vi "CFG File Editor.vi"(0 "Parameters In":T1[](array[typedef]), 11 "error in (no error)":errorcluster) -> (4 "Parameters Out":T1[](array[typedef]), 8 "Cancelled":bool, 15 "error out":errorcluster)   [LabVIEW 2012]
uses:
  Type Defs/CFG Key Cluster.ctl
  Type Defs/CFG Tag Type Enum.ctl
panel:
  in  "DAQmx Terminal":tag
  in  "DAQmx Channel":tag
  in  "Exit":bool
  in  "I32":i32
  in  "VISA resource name":refnum<visa-resource-name>
  in  "VISA Rsrc":refnum<visa-resource-name>
  in  "String":string
  in  "Ring":u16(ring) items=["Yaw/Brake ATP", "Yaw/Brake Integration/Endurance", "Pitch/Roll ATP", "Pitch/Roll Integration/Endurance", "Control Stand"]
  in  "Path":path
  in  "BOOL":bool
  in  "DBL":dbl min=1.0 max=160.0 step=1.0
  in  "Cancel":bool
  out "Status":string="Initialize"
  in  "Tree":string(tree)
  # "Configuration"
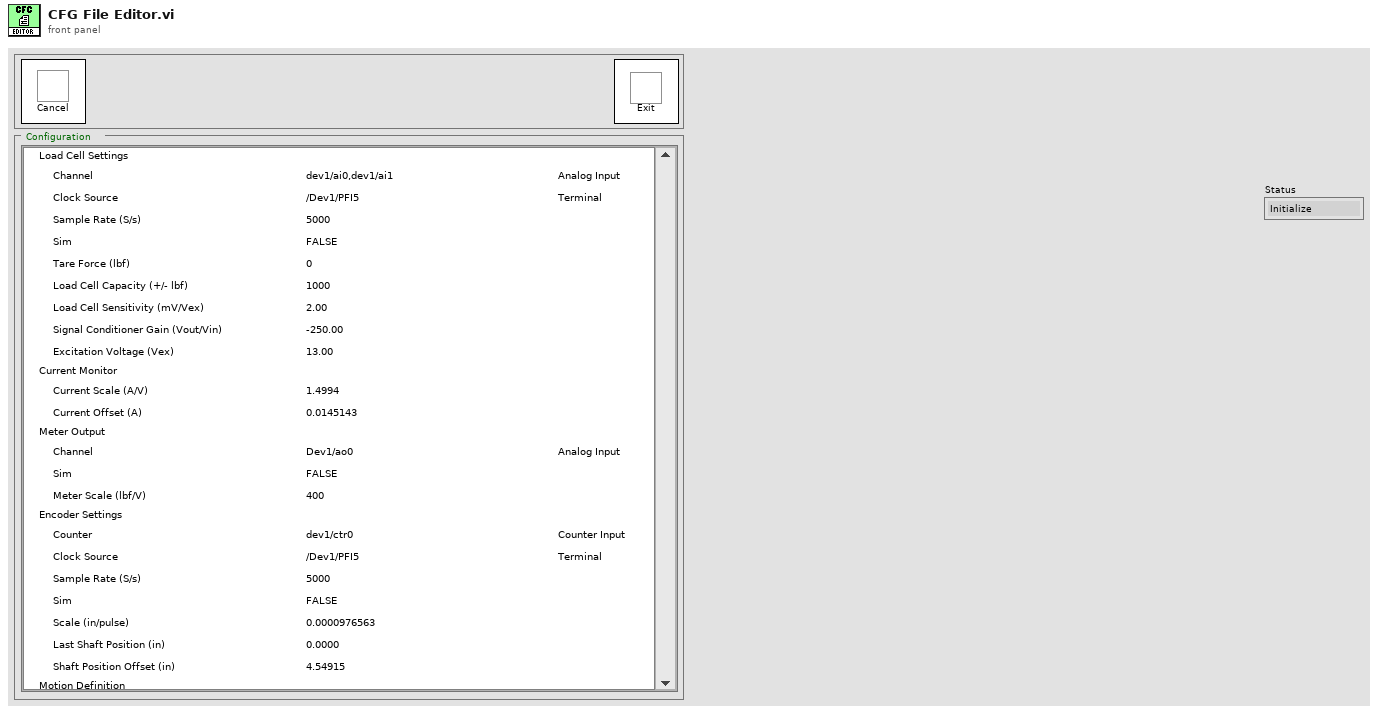
[diagram p1: front panel]
types:
  T1 = typedef "CFG Key Cluster.ctl" = cluster{"Strings []":string[], "Disabled Items []":i32[], "Value":variant, "Format String":string, "Tag":string, "Type":T2, "Section":string, " Ctl Ref":refnum<vi>, "Data Range":cluster{"Minimum":dbl, "Maximum":dbl, "Increment":dbl}, "Unit":string, "Special Instructions":string, "Delimiter(s)":string, "Dimensions":i32, "Element Type":T2, "Array Value String":string}
  T2 = typedef "CFG Tag Type Enum.ctl" = enum16{"Digital", "Slide", "Enum", "Boolean", "String", "Path", "Array", "VISAResourceName", "DAQmxName", "Cluster"}
  T3 = enum32{"existing file", "new file", "new or existing file", "existing dir", "new dir", "new or existing dir", "existing file (use LLBs)", "new file (use LLBs)", "new or existing file (use LLBs)", "new or existing file or directory (use LLBs)", "existing dir (use LLBs)", "new dir (use LLBs)", "new or existing dir (use LLBs)", "existing file or dir", "new file or dir", "new or existing file or dir", "existing file or dir (use LLBs)", "new file or dir (use LLBs)"}
  T4 = cluster{"Minimum":dbl, "Maximum":dbl, "Increment":dbl}
  T5 = typedef "LVPositionTypeDef.ctl" = cluster{"Left":i32, "Top":i32}
  T6 = typedef "CFG DAQmx Type Enum.ctl" = enum16{"Analog Input", "Analog Output", "Digital Input", "Digital Output", "Counter Input", "Counter Output", "Terminal", ""}
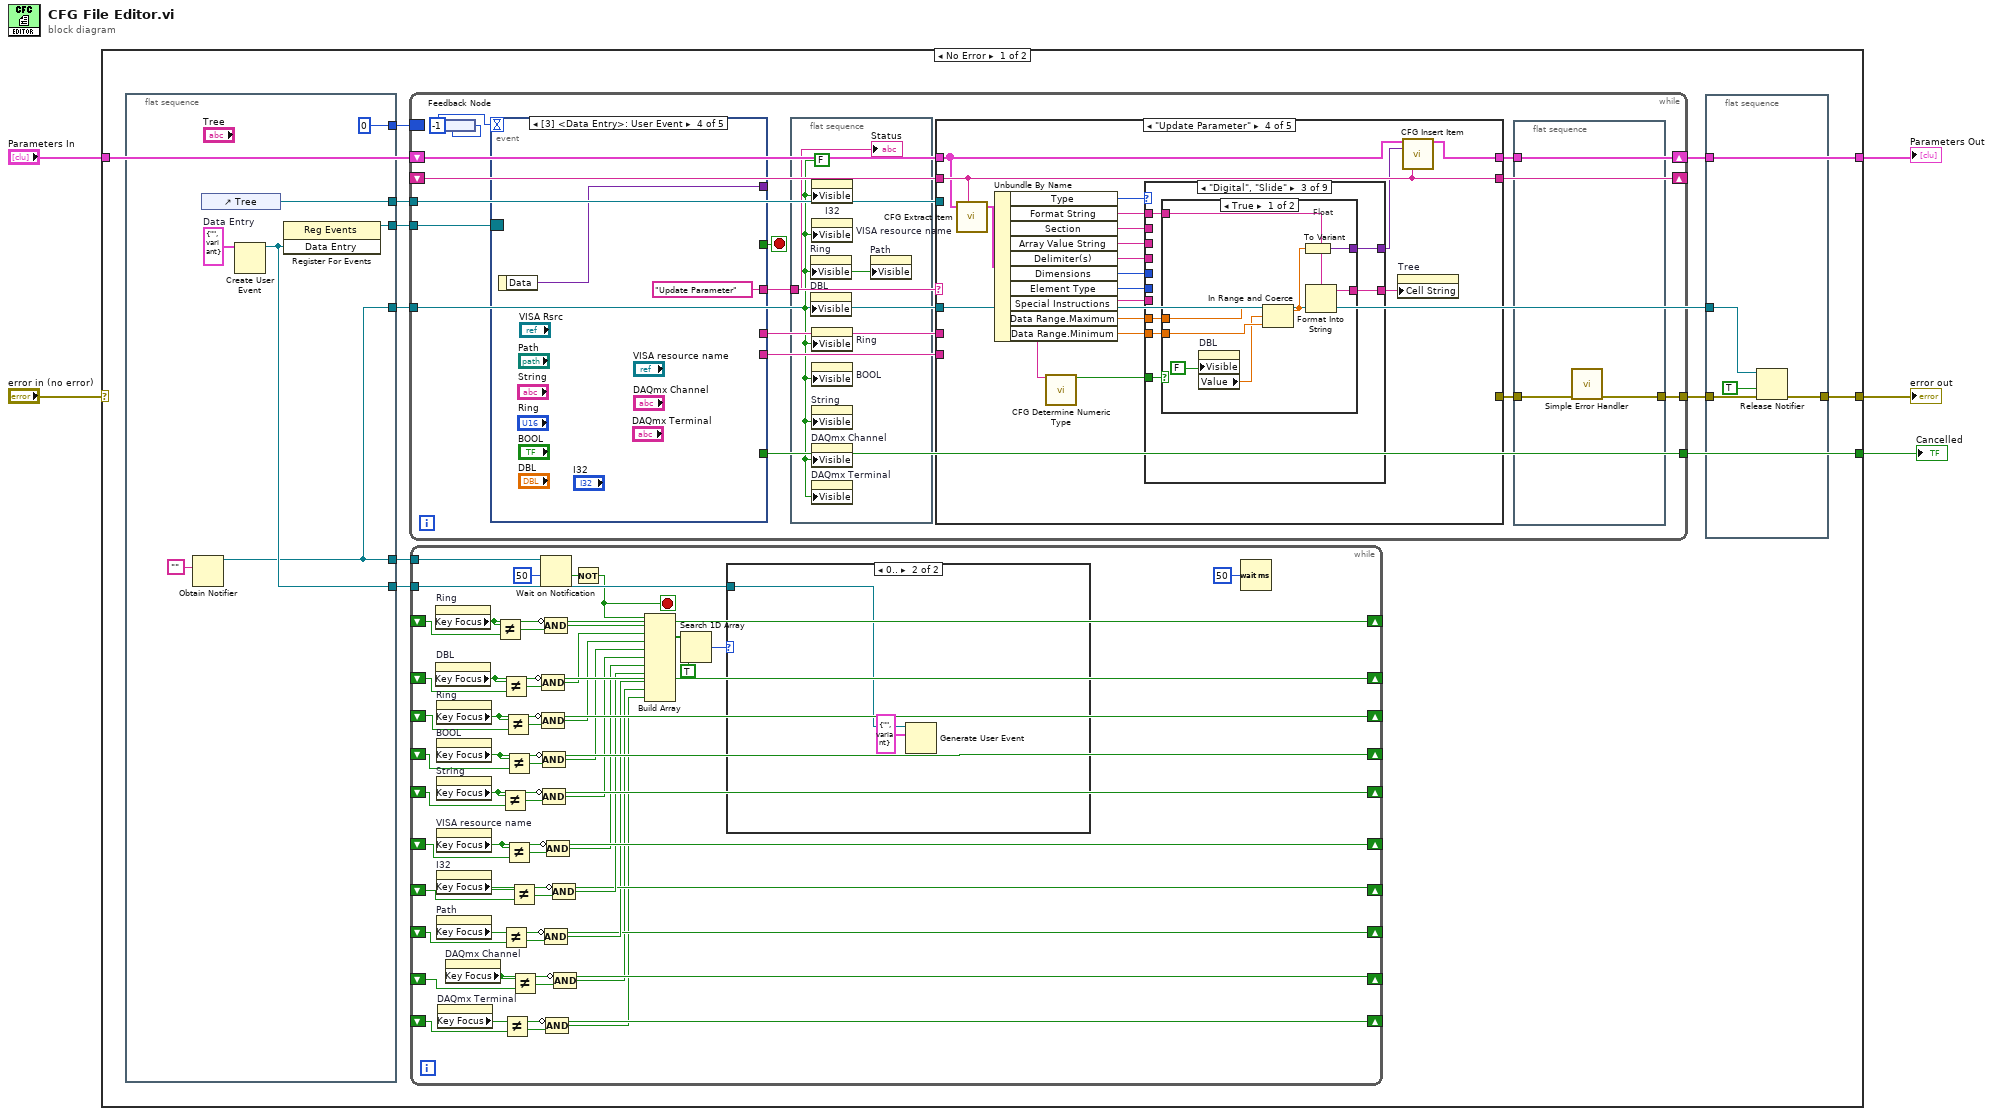
[diagram p0: block diagram]
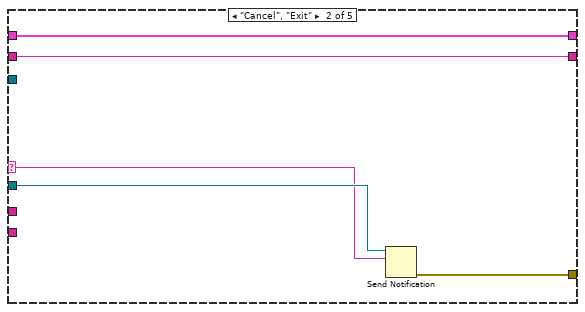
[diagram p4: hidden frame]
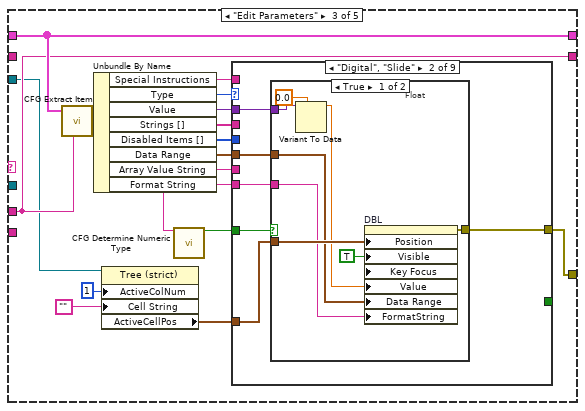
[diagram p5: hidden frame]
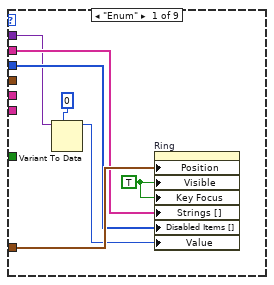
[diagram p6: hidden frame]
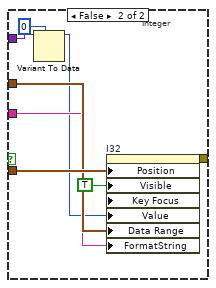
[diagram p7: hidden frame]
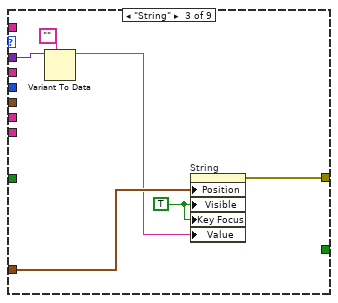
[diagram p8: hidden frame]
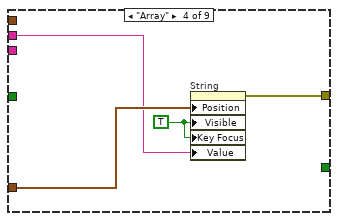
[diagram p9: hidden frame]
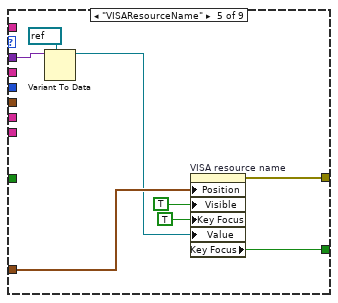
[diagram p10: hidden frame]
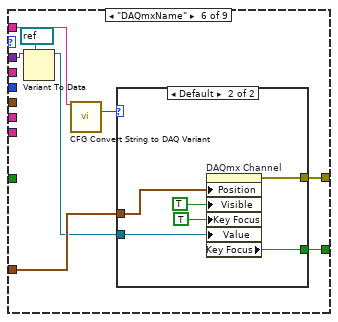
[diagram p11: hidden frame]
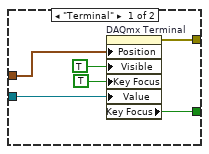
[diagram p12: hidden frame]
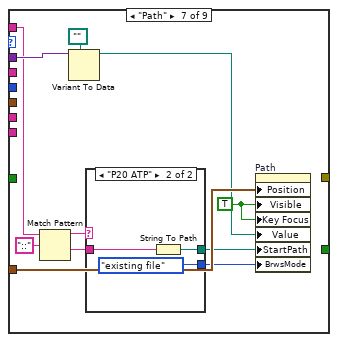
[diagram p13: hidden frame]
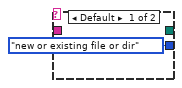
[diagram p14: hidden frame]
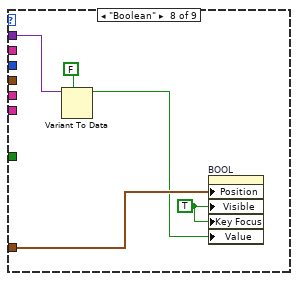
[diagram p15: hidden frame]
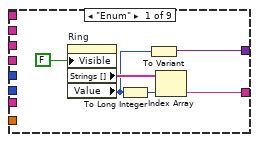
[diagram p17: hidden frame]
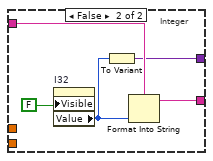
[diagram p19: hidden frame]
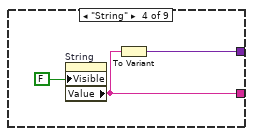
[diagram p20: hidden frame]
diagram:
  n1 = case shown="No Error" "error in (no error)" {
    selector: "error in (no error)" -> [_ w313]
    tunnel: [w14 w312] -> w5
    tunnel: "Parameters In" -> [w13 w312]
    tunnel: [w7 w313] -> w2
    tunnel: [w12 _] -> w1
    frame No Error {
      n2 = flat-sequence {
        tunnel: [0] -> w16
        tunnel: [w77] -> w15
        tunnel: [w75] -> w11
        tunnel: [w74] -> w10
        tunnel: [w72] -> w9
        tunnel: [w72] -> w6
        frame #0 {
          w76 = cluster{"Item":string, "Data":variant} {"Item"="", "Data"=variant}  # Data Entry
          n3 = Obtain Notifier(notification data type="") -> (notifier out=w72:refnum<notifier>)  [unwired: 2 in, 3 out]
          n4 = control-ref of="Tree"() -> (w77:refnum<vi>)
          n5 = Create User Event(user event datatype=w76) -> (user event=w74:refnum<user-event>)  [unwired: 1 in, 1 out]
          n6 = register-events(w74) -> (reference out=w75:refnum<event-registration>)  [unwired: 2 in, 1 out]
        }
      }
      n7 = while {
        tunnel: w15 -> [w90]
        shift-right: [w84] -> w14
        shift-left: w13 -> [w88]
        shift-right: [w87] -> _
        shift-left: _ -> [w86]
        tunnel: [w82] -> w8
        tunnel: [w81] -> w12
        tunnel: w11 -> [w80]
        tunnel: w6 -> [w79]
        border: w16 -> [_]
        stop <- w85 stop-if-true
        n8 = feedback-in #1(-1) -> ()
        n9 = feedback #1() -> (w93:i32)
        n10 = event shown="[3] <Data Entry>: User Event" {
          selector: w80 -> [_ _ _ _ _]
          dyn-events: _ -> [_ _ _ _ _]
          timeout: w93 -> [_ _ _ _ _]
          tunnel: [w297 "Initialize" ("Tag") w305 "Update Parameter" ("Tag") "Update Parameter" ("Tag")] -> w92
          tunnel: [w302 _ _ _ _] -> w89
          tunnel: [_ _ TRUE ("Exit") _ _] -> w85
          tunnel: [w300 _ _ _ _] -> w83
          tunnel: [_ _ "Cancel" _ _] -> w81
          tunnel: [_ _ _ w309 _] -> _
          event "Tree": Double Click {
            n11 = event-data() -> ("CtlRef"=w303:refnum<vi>, "Tag"=w302:string)  [unwired: 1 out]
            n12 = property on="Property Node" class="Tree (strict)"(reference=w303, "Active Item Tag"=w302, "ActiveColNum"=0 ("Active Cell:Active Column Number")) -> ("Indent Level"=w298:i32, "Cell String"=w300:string)  [unwired: 1 in, 2 out]
            n13 = Index Array(array=string[] ["", "Edit Parameters"], index=w298) -> (element=w297:string)
          }
          event Timeout {
            n14 = event-data() -> ()  [unwired: 2 out]
          }
          event "Cancel", "Exit": Value Change {
            n15 = event-data() -> ("CtlRef"=w306:refnum<vi>)  [unwired: 1 out]
            n16 = property class="Bool"(reference=w306) -> ("Label.Text"=w305:string)  [unwired: 1 in, 2 out]
          }
          event User Event {
            n17 = event-data() -> ("Data"=w309:variant)  [unwired: 1 out]
          }
          event "DBL", "BOOL", "String", "Path", "Ring", "I32": Value Change {
            n18 = event-data() -> ()  [unwired: 7 out]
          }
        }
        n19 = flat-sequence {
          tunnel: w92 -> [w98]
          frame #0 {
            w97 = FALSE ("Visible")
            n20 = property on="Ring" class="Ring (strict)"("Visible"=w97) -> ()  [unwired: 2 in, 2 out]
            n21 = property on="DBL" class="DigNum (strict)"("Visible"=w97) -> ()  [unwired: 2 in, 2 out]
            n22 = property on="I32" class="DigNum (strict)"("Visible"=w97) -> ()  [unwired: 2 in, 2 out]
            n23 = property on="VISA resource name" class="VISAName"("Visible"=w97) -> ()  [unwired: 2 in, 2 out]
            n24 = property on="Ring" class="Ring (strict)"("Visible"=w97) -> ()  [unwired: 2 in, 2 out]
            n25 = property on="BOOL" class="Bool (strict)"("Visible"=w97) -> ()  [unwired: 2 in, 2 out]
            n26 = property on="String" class="Str"("Visible"=w97) -> ()  [unwired: 2 in, 2 out]
            n27 = property on="DAQmx Channel" class="DAQmxName"("Visible"=w97) -> ()  [unwired: 2 in, 2 out]
            n28 = property on="DAQmx Terminal" class="DAQmxName"("Visible"=w97) -> ()  [unwired: 2 in, 2 out]
            n29 = property on="Path" class="Path"("Visible"=w97) -> ()  [unwired: 2 in, 2 out]
            "Status" <- w98
          }
        }
        n30 = case shown="\"Update Parameter\"" w92 {
          selector: w92 -> [_ w101 _ _ _]
          tunnel: [_ w103 w108 _ w295] -> w91
          tunnel: w90 -> [_ _ w113 _ w294]
          tunnel: w89 -> [_ _ w118 _ _]
          tunnel: [w100 w105 w119 w222 w293] -> w84
          tunnel: w88 -> [w100 w105 w119 w223 w293]
          tunnel: [w99 w104 w118 w225 w296] -> w87
          tunnel: w86 -> [w99 w104 _ w225 w296]
          tunnel: w83 -> [_ _ _ _ _]
          tunnel: w79 -> [_ w102 _ _ _]
          frame Default {
          }
          frame "Cancel", "Exit" {
            n31 = Send Notification(notification=w101, notifier=w102) -> (error out=w103:errorcluster)  [unwired: 1 in, 1 out]
          }
          frame "Edit Parameters" {
            n32 = call "CFG Extract Item.vi"("Parameters"=w119, "Tag"=w118) -> ("Key Cluster"=w117:T1)  [unwired: 7 out]
            n33 = Unbundle By Name(w117) -> ("Special Instructions"=w107:string, "Type"=w122:T2, "Value"=w121:variant, "Strings []"=w120:string[], "Disabled Items []"=w116:i32[], "Data Range"=w115:T4, "Array Value String"=w106:string, "Format String"=w110:string)
            n34 = property on="Property Node" class="Tree (strict)"(reference=w113, "ActiveColNum"=1 ("Active Cell:Active Column Number"), "Cell String"="") -> ("ActiveCellPos"=w114:T5)  [unwired: 1 in, 2 out]
            n35 = call "CFG Determine Numeric Type.vi"("Format String"=w110) -> ("Float"=w109:bool)  [unwired: 14 out]
            n36 = case shown="\"Digital\", \"Slide\"" w122 {
              tunnel: w114 -> [w129 w135 w157 w161 w169 w177 w200 w209 _]
              tunnel: w121 -> [w125 w132 w155 _ w167 w176 w198 w207 _]
              tunnel: w120 -> [w127 _ _ _ _ _ _ _ _]
              tunnel: w116 -> [w126 _ _ _ _ _ _ _ _]
              tunnel: w115 -> [_ w134 _ _ _ _ _ _ _]
              tunnel: w110 -> [_ w133 _ _ _ _ _ _ _]
              tunnel: [_ w131 w152 w159 w162 w172 _ _ _] -> w108
              tunnel: [_ _ _ _ w163 w173 _ _ _] -> _
              tunnel: w109 -> [_ w130 _ _ _ _ _ _ _]
              tunnel: w107 -> [_ _ _ _ _ w171 w195 _ _]
              tunnel: w106 -> [_ _ _ w158 _ _ _ _ _]
              frame "Enum" {
                w128 = TRUE ("Visible")
                n37 = Variant To Data(type=i16 0 ("Ring"), Variant=w125) -> (data=w123:i16)  [unwired: 1 in, 1 out]
                n38 = property on="Ring" class="Ring (strict)"("Position"=w129, "Visible"=w128, "Key Focus"=w128, "Strings []"=w127, "Disabled Items []"=w126, "Value"=w123) -> ()  [unwired: 2 in, 2 out]
              }
              frame "Digital", "Slide" {
                n39 = case shown="True" w130 {
                  tunnel: w135 -> [w143 w151]
                  tunnel: w134 -> [w141 w149]
                  tunnel: w133 -> [w140 w148]
                  tunnel: w132 -> [w139 w147]
                  tunnel: [w136 w144] -> w131
                  frame True {
                    w142 = TRUE ("Visible")
                    # "Float"
                    n40 = Variant To Data(type=0.0 ("DBL"), Variant=w139) -> (data=w137:dbl)  [unwired: 1 in, 1 out]
                    n41 = property on="DBL" class="DigNum (strict)"("Position"=w143, "Visible"=w142, "Key Focus"=w142, "Value"=w137, "Data Range"=w141, "FormatString"=w140) -> (error out=w136:errorcluster)  [unwired: 2 in, 1 out]
                  }
                  frame False {
                    w150 = TRUE ("Visible")
                    # "Integer"
                    n42 = Variant To Data(type=0 ("DBL"), Variant=w147) -> (data=w145:i32)  [unwired: 1 in, 1 out]
                    n43 = property on="I32" class="DigNum (strict)"("Position"=w151, "Visible"=w150, "Key Focus"=w150, "Value"=w145, "Data Range"=w149, "FormatString"=w148) -> (error out=w144:errorcluster)  [unwired: 2 in, 1 out]
                  }
                }
              }
              frame "String" {
                w156 = TRUE ("Visible")
                n44 = Variant To Data(type="" ("DBL"), Variant=w155) -> (data=w153:string)  [unwired: 1 in, 1 out]
                n45 = property on="String" class="Str"("Position"=w157, "Visible"=w156, "Key Focus"=w156, "Value"=w153) -> (error out=w152:errorcluster)  [unwired: 2 in, 1 out]
              }
              frame "Array" {
                w160 = TRUE ("Visible")
                n46 = property on="String" class="Str"("Position"=w161, "Visible"=w160, "Key Focus"=w160, "Value"=w158) -> (error out=w159:errorcluster)  [unwired: 2 in, 1 out]
              }
              frame "VISAResourceName" {
                n47 = Variant To Data(type=refnum<visa-resource-name> refnum ("VISA resource name"), Variant=w167) -> (data=w166:refnum<visa-resource-name>)  [unwired: 1 in, 1 out]
                n48 = property on="VISA resource name" class="VISAName"("Position"=w169, "Visible"=TRUE, "Key Focus"=TRUE, "Value"=w166) -> (error out=w162:errorcluster, "Key Focus"=w163:bool)  [unwired: 2 in, 1 out]
              }
              frame "DAQmxName" {
                n49 = Variant To Data(type=refnum<visa-resource-name> refnum ("VISA resource name"), Variant=w176) -> (data=w175:refnum<visa-resource-name>)  [unwired: 1 in, 1 out]
                n50 = call "CFG Convert String to DAQ Variant.vi"("Special Instructions"=w171) -> ("DAQmx Type"=w170:T6)  [unwired: 3 in, 11 out]
                n51 = case shown="Default" w170 {
                  tunnel: w177 -> [w183 w189]
                  tunnel: w175 -> [w181 w187]
                  tunnel: [w179 w185] -> w173
                  tunnel: [w178 w184] -> w172
                  frame "Terminal" {
                    n52 = property on="DAQmx Terminal" class="DAQmxName"("Position"=w183, "Visible"=TRUE, "Key Focus"=TRUE, "Value"=w181) -> (error out=w178:errorcluster, "Key Focus"=w179:bool)  [unwired: 2 in, 1 out]
                  }
                  frame Default {
                    n53 = property on="DAQmx Channel" class="DAQmxName"("Position"=w189, "Visible"=TRUE, "Key Focus"=TRUE, "Value"=w187) -> (error out=w184:errorcluster, "Key Focus"=w185:bool)  [unwired: 2 in, 1 out]
                  }
                }
              }
              frame "Path" {
                w199 = TRUE ("Visible")
                n54 = Match Pattern(string=w195, regular expression="::") -> (before substring=w193:string, after substring=w192:string)  [unwired: 3 out]
                n55 = Variant To Data(type=path "" ("DBL"), Variant=w198) -> (data=w196:path)  [unwired: 1 in, 1 out]
                n56 = case shown="\"P20 ATP\"" w193 {
                  tunnel: w192 -> [_ w203]
                  tunnel: [_ w204] -> w191
                  tunnel: [T3."new or existing file or dir" ("Browse Options:Selection Mode") T3."existing file" ("Browse Options:Selection Mode")] -> w190
                  frame Default {
                  }
                  frame "P20 ATP" {
                    n57 = String To Path(string=w203) -> (path=w204:path)
                  }
                }
                n58 = property on="Path" class="Path"("Position"=w200, "Visible"=w199, "Key Focus"=w199, "Value"=w196, "StartPath"=w191, "BrwsMode"=w190) -> ()  [unwired: 2 in, 2 out]
              }
              frame "Boolean" {
                w208 = TRUE ("Visible")
                n59 = Variant To Data(type=FALSE ("Visible"), Variant=w207) -> (data=w205:bool)  [unwired: 1 in, 1 out]
                n60 = property on="BOOL" class="Bool (strict)"("Position"=w209, "Visible"=w208, "Key Focus"=w208, "Value"=w205) -> ()  [unwired: 2 in, 2 out]
              }
              frame "Cluster" {
              }
            }
          }
          frame "Update Parameter" {
            n61 = call "CFG Extract Item.vi"("Parameters"=w223, "Tag"=w225) -> ("Key Cluster"=w226:T1)  [unwired: 7 out]
            n62 = Unbundle By Name(w226) -> ("Type"=w220:T2, "Format String"=w219:string, "Section"=w217:string, "Array Value String"=w215:string, "Delimiter(s)"=w214:string, "Dimensions"=w213:i32, "Element Type"=w212:T2, "Special Instructions"=w216:string, "Data Range.Maximum"=w211:dbl, "Data Range.Minimum"=w210:dbl)
            n63 = call "CFG Determine Numeric Type.vi"("Format String"=w219) -> ("Float"=w218:bool)  [unwired: 14 out]
            n64 = case shown="\"Digital\", \"Slide\"" w220 {
              tunnel: [w230 _ w238 w252 w260 w262 w269 w282 w291] -> w224
              tunnel: w219 -> [_ _ w237 _ _ _ _ _ _]
              tunnel: [w228 _ w236 w253 w259 w264 w271 w283 w289] -> w221
              tunnel: w218 -> [_ _ w235 _ w256 _ _ _ _]
              tunnel: w217 -> [_ _ _ _ _ _ _ w280 _]
              tunnel: w216 -> [_ _ _ _ _ _ w268 w278 _]
              tunnel: w215 -> [_ _ _ _ _ _ _ _ _]
              tunnel: w214 -> [_ _ _ _ w255 _ _ _ _]
              tunnel: w213 -> [_ _ _ _ w258 _ _ _ _]
              tunnel: w212 -> [_ _ _ _ w257 _ _ _ _]
              tunnel: w211 -> [_ _ w234 _ _ _ _ _ _]
              tunnel: w210 -> [_ _ w233 _ _ _ _ _ _]
              frame "Enum" {
                n65 = property on="Ring" class="Ring (strict)"("Visible"=FALSE) -> ("Strings []"=w231:string[], "Value"=w227:u16)  [unwired: 2 in, 2 out]
                n66 = To Long Integer(number=w227) -> (32bit integer=w229:i32)
                n67 = To Variant(anything=w227) -> (Variant=w228:variant)
                n68 = Index Array(array=w231, index=w229) -> (element=w230:string)
              }
              frame "Cluster" {
              }
              frame "Digital", "Slide" {
                n69 = case shown="True" w235 {
                  tunnel: [w245 w250] -> w238
                  tunnel: w237 -> [w244 w249]
                  tunnel: [w243 w247] -> w236
                  tunnel: w234 -> [w242 _]
                  tunnel: w233 -> [w241 _]
                  frame True {
                    # "Float"
                    n70 = property on="DBL" class="DigNum (strict)"("Visible"=FALSE) -> ("Value"=w239:dbl)  [unwired: 2 in, 2 out]
                    n71 = In Range and Coerce(upper limit=w242, x=w239, lower limit=w241) -> (coerced(x)=w240:dbl)  [unwired: 1 out]
                    n72 = To Variant(anything=w240) -> (Variant=w243:variant)
                    n73 = Format Into String(format string=w244, w240) -> (resulting string=w245:string)  [unwired: 2 in, 1 out]
                  }
                  frame False {
                    # "Integer"
                    n74 = property on="I32" class="DigNum (strict)"("Visible"=FALSE) -> ("Value"=w248:i32)  [unwired: 2 in, 2 out]
                    n75 = To Variant(anything=w248) -> (Variant=w247:variant)
                    n76 = Format Into String(format string=w249, w248) -> (resulting string=w250:string)  [unwired: 2 in, 1 out]
                  }
                }
              }
              frame "String" {
                n77 = property on="String" class="Str"("Visible"=FALSE) -> ("Value"=w252:string)  [unwired: 2 in, 2 out]
                n78 = To Variant(anything=w252) -> (Variant=w253:variant)
              }
              frame "Array" {
                n79 = property on="String" class="Str"("Visible"=FALSE) -> ("Value"=w260:string)  [unwired: 2 in, 2 out]
                n80 = call "CFG Build Array Value.vi"("Value String"=w260, "Delimiter(s)"=w255, "Dimensions"=w258, "Element Type"=w257, "Float"=w256) -> ("Variant"=w259:variant)  [unwired: 1 in, 9 out]
              }
              frame "VISAResourceName" {
                n81 = property on="VISA resource name" class="VISAName"("Visible"=FALSE) -> ("Value"=w263:refnum<visa-resource-name>)  [unwired: 2 in, 2 out]
                n82 = Concatenate Strings(w263) -> (w262:string)
                n83 = To Variant(anything=w263) -> (Variant=w264:variant)
              }
              frame "DAQmxName" {
                n84 = call "CFG Convert String to DAQ Variant.vi"("Special Instructions"=w268) -> ("DAQmx Type"=w267:T6, "Channel Signal Type"=w266:i32)  [unwired: 3 in, 10 out]
                n85 = case shown="Default" w267 {
                  tunnel: [w273 w274] -> w270
                  tunnel: w266 -> [_ _]
                  frame Default {
                    n86 = property on="DAQmx Channel" class="DAQmxName"("Visible"=FALSE) -> ("Value"=w273:string)  [unwired: 2 in, 2 out]
                  }
                  frame "Terminal" {
                    n87 = property on="DAQmx Terminal" class="DAQmxName"("Visible"=FALSE) -> ("Value"=w274:string)  [unwired: 2 in, 2 out]
                  }
                }
                n88 = To Variant(anything=w270) -> (Variant=w271:variant)
                n89 = Concatenate Strings(w270) -> (w269:string)
              }
              frame "Path" {
                n90 = property on="Path" class="Path"("Visible"=FALSE) -> ("Value"=w281:path)  [unwired: 2 in, 2 out]
                n91 = Match Pattern(string=w278, regular expression="::") -> (before substring=w277:string)  [unwired: 4 out]
                n92 = case shown="\"P20 ATP\"" w277 {
                  tunnel: w281 -> [w285 w288]
                  tunnel: w280 -> [_ w287]
                  tunnel: [w285 w286] -> w279
                  frame Default {
                  }
                  frame "P20 ATP" {
                    n93 = call "CFG Handle P20 ATP Sequence Paths.vi"("Path"=w288, "Section"=w287) -> ("ATP Relative Path"=w286:path)  [unwired: 1 in, 12 out]
                  }
                }
                n94 = To Variant(anything=w279) -> (Variant=w283:variant)
                n95 = Path To String(path=w279) -> (string=w282:string)
              }
              frame "Boolean" {
                n96 = property on="BOOL" class="Bool (strict)"("Visible"=FALSE) -> ("Value"=w290:bool)  [unwired: 2 in, 2 out]
                n97 = Format Into String(w290) -> (resulting string=w291:string)  [unwired: 3 in, 1 out]
                n98 = To Variant(anything=w290) -> (Variant=w289:variant)
              }
            }
            n99 = property on="Tree" class="Tree (strict)"("Cell String"=w224) -> ()  [unwired: 2 in, 2 out]
            n100 = call "CFG Insert Item.vi"("Parameters"=w223, "Value"=w221, "Tag"=w225) -> ("Parameters"=w222:T1[])  [unwired: 1 in, 11 out]
          }
          frame "Initialize" {
            n101 = call "CFG Load Tree.vi"("Tree"=w294, "Parameters In"=w293) -> ("error Out"=w295:errorcluster)  [unwired: 1 in, 12 out]
          }
        }
        n102 = flat-sequence {
          tunnel: w91 -> [w96]
          tunnel: w84 -> [_]
          tunnel: [w95] -> w82
          frame #0 {
            n103 = call <vilib>:"Simple Error Handler.vi"("error in (no error)"=w96) -> ("error out"=w95:errorcluster)  [unwired: 4 in, 4 out]
          }
        }
      }
      n104 = while {
        shift-right: [w60] -> _
        shift-left: _ -> [w65]
        shift-right: [w53] -> _
        shift-left: _ -> [w64]
        shift-right: [w54] -> _
        shift-left: _ -> [w63]
        shift-right: [w55] -> _
        shift-left: _ -> [w62]
        shift-right: [w56] -> _
        shift-left: _ -> [w61]
        tunnel: w10 -> [w44]
        shift-right: [w39] -> _
        shift-left: _ -> [w40]
        shift-right: [w34] -> _
        shift-left: _ -> [w37]
        tunnel: w9 -> [w32]
        shift-right: [w25] -> _
        shift-left: _ -> [w27]
        shift-right: [w20] -> _
        shift-left: _ -> [w21]
        shift-right: [w19] -> _
        shift-left: _ -> [w24]
        stop <- w30 stop-if-true
        n105 = property on="Ring" class="Ring (strict)"() -> ("Key Focus"=w60:bool)  [unwired: 2 in, 2 out]
        n106 = property on="DBL" class="DigNum (strict)"() -> ("Key Focus"=w53:bool)  [unwired: 2 in, 2 out]
        n107 = property on="Ring" class="Ring (strict)"() -> ("Key Focus"=w54:bool)  [unwired: 2 in, 2 out]
        n108 = property on="BOOL" class="Bool (strict)"() -> ("Key Focus"=w55:bool)  [unwired: 2 in, 2 out]
        n109 = property on="String" class="Str"() -> ("Key Focus"=w56:bool)  [unwired: 2 in, 2 out]
        n110 = property on="VISA resource name" class="VISAName"() -> ("Key Focus"=w39:bool)  [unwired: 2 in, 2 out]
        n111 = property on="I32" class="DigNum (strict)"() -> ("Key Focus"=w34:bool)  [unwired: 2 in, 2 out]
        n112 = property on="Path" class="Path"() -> ("Key Focus"=w25:bool)  [unwired: 2 in, 2 out]
        n113 = property on="DAQmx Terminal" class="DAQmxName"() -> ("Key Focus"=w19:bool)  [unwired: 2 in, 2 out]
        n114 = property on="DAQmx Channel" class="DAQmxName"() -> ("Key Focus"=w20:bool)  [unwired: 2 in, 2 out]
        n115 = Not Equal?(x=w60, y=w65) -> (x != y?=w33:bool)
        n116 = Not Equal?(x=w56, y=w61) -> (x != y?=w57:bool)
        n117 = Not Equal?(x=w53, y=w64) -> (x != y?=w52:bool)
        n118 = Not Equal?(x=w25, y=w27) -> (x != y?=w28:bool)
        n119 = Not Equal?(x=w19, y=w24) -> (x != y?=w23:bool)
        n120 = Not Equal?(x=w54, y=w63) -> (x != y?=w59:bool)
        n121 = Not Equal?(x=w55, y=w62) -> (x != y?=w58:bool)
        n122 = Not Equal?(x=w39, y=w40) -> (x != y?=w41:bool)
        n123 = Not Equal?(x=w34, y=w37) -> (x != y?=w36:bool)
        n124 = Not Equal?(x=w20, y=w21) -> (x != y?=w22:bool)
        n125 = Wait on Notification(notifier=w32, timeout in ms (-1)=50) -> (timed out?=w31:bool)  [unwired: 1 in, 4 out]
        n126 = Compound Arithmetic op=AND(invert w53, w52) -> (w50:bool)
        n127 = Compound Arithmetic op=AND(invert w54, w59) -> (w49:bool)
        n128 = Compound Arithmetic op=AND(invert w55, w58) -> (w48:bool)
        n129 = Compound Arithmetic op=AND(invert w56, w57) -> (w47:bool)
        n130 = Compound Arithmetic op=AND(invert w60, w33) -> (w51:bool)
        n131 = Compound Arithmetic op=AND(invert w25, w28) -> (w26:bool)
        n132 = Compound Arithmetic op=AND(invert w19, w23) -> (w17:bool)
        n133 = Compound Arithmetic op=AND(invert w39, w41) -> (w38:bool)
        n134 = Compound Arithmetic op=AND(invert w34, w36) -> (w35:bool)
        n135 = Compound Arithmetic op=AND(invert w20, w22) -> (w18:bool)
        n136 = Not(x=w31) -> (.not. x?=w30:bool)
        n137 = Build Array(w30, w51, w50, w49, w48, w47, w38, w35, w26, w18, w17) -> (w46:bool[])
        n138 = Search 1D Array(1D array=w46, element=TRUE) -> (index of element=w45:i32)  [unwired: 1 out]
        n139 = case shown="0.." w45 {
          tunnel: w44 -> [_ w67]
          frame Default {
          }
          frame 0.. {
            n140 = Generate User Event(user event=w67, event data cluster=cluster{"Item":string, "Data":variant} {"Item"="", "Data"=variant} ("event data")) -> ()  [unwired: 1 in, 2 out]
          }
        }
        n141 = Wait (ms)(milliseconds to wait=u32 50) -> ()  [unwired: 1 out]
      }
      n142 = flat-sequence {
        tunnel: w14 -> [_]
        tunnel: w6 -> [w69]
        tunnel: w8 -> [w71]
        tunnel: [w70] -> w7
        frame #0 {
          n143 = Release Notifier(notifier=w69, force destroy? (F)=TRUE, error in (no error)=w71) -> (error out=w70:errorcluster)  [unwired: 2 out]
        }
      }
    }
    frame Error {
    }
  }
  "Parameters Out" <- w5
  "error out" <- w2
  "Cancelled" <- w1
